vi "load_manual.vi"(8 "error in (no error)":errorcluster) -> (0 "error out":errorcluster, 2 "replaced_action(s)":bool, 3 "manual_actions out":variant)   [LabVIEW 2015, in "example_02.lvlib"]
doc: "load_manual.vi will assign manual steps as variant attributes to an empty variant. An indicator is provided if actions are replaced (e.g. a duplicate key)."
uses:
  example_02.lvlib
  <userlib>/antonio-alexander/lv-recipe-machine/public/_controls/step.ctl
  <userlib>/antonio-alexander/lv-recipe-machine/public/_controls/vi_reference_type.ctl
  _controls/steps_actions.ctl
  <userlib>/antonio-alexander/lv-recipe-machine/public/_controls/vi_reference_manual_action.ctl
  <userlib>/antonio-alexander/lv-recipe-machine/lv-recipe-machine.lvlib
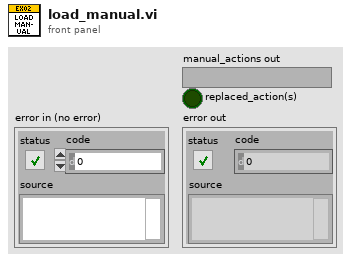
[diagram p1: front panel]
types:
  T1 = typedef "lv-recipe-machine.lvlib/vi_reference_type.ctl" = enum16{"<vi_reference_type>", "manual_action", "auto_step", "auto_criteria", "auto_transition", "auto_launcher", "<null>"}
  T2 = typedef "lv-recipe-machine.lvlib/step.ctl" = cluster{"name":string, "vi_reference":variant}
  T3 = typedef "lv-recipe-machine.lvlib/vi_reference_manual_action.ctl" = refnum<vi>
  T4 = typedef "example_02.lvlib/steps_actions.ctl" = enum16{"<steps_actions>", "auto_initialize", "auto_first_name", "auto_last_name", "criteria_", "transition", "launch_", "<null>"}
  T5 = cluster{"vi_reference_type":T1, "manual_action":T3}
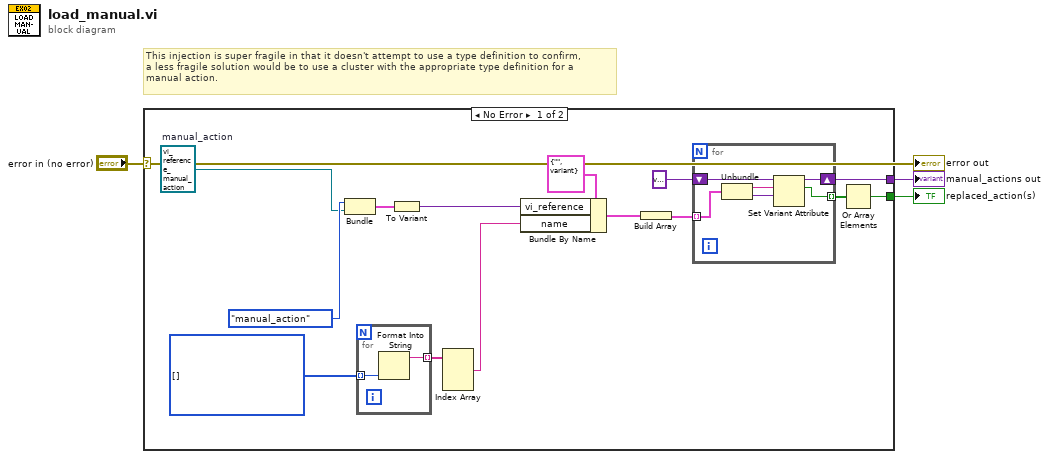
[diagram p0: block diagram]
diagram:
  # "This injection is super fragile in that it doesn't attempt to use a type definition to confirm,\na less fragile solution would be to use a cluster with the appropriate type definition for a\nmanual action."
  n1 = case shown="No Error" "error in (no error)" {
    tunnel: [w17 _] -> w3
    tunnel: [w14 _] -> w2
    frame No Error {
      w6 = T3 refnum  # manual_action
      w9 = T4[] [] items=["<steps_actions>", "auto_initialize", "auto_first_name", "auto_last_name", "criteria_", "transition", "launch_", "<null>"]
      n2 = Bundle("vi_reference_type"=vi_reference_type."manual_action", "manual_action"=w6) -> (w11:T5)  [unwired: 1 in]
      n3 = for {
        tunnel: w9 -> [w19] mode=indexing
        tunnel: [w18] -> w8 mode=indexing
        n4 = Format Into String(w19) -> (resulting string=w18:string)  [unwired: 3 in, 1 out]
      }
      n5 = To Variant(anything=w11) -> (Variant=w12:variant)
      n6 = Index Array(array=w8) -> (element #1=w7:string)  [unwired: 3 in, 2 out]
      n7 = Bundle By Name(cluster=T2 {"name"="", "vi_reference"=variant(refnum<vi> refnum)} ("step"), "vi_reference"=w12, "name"=w7) -> (w4:T2)
      n8 = Build Array(w4) -> (w16:T2[])
      n9 = for {
        tunnel: w16 -> [w23] mode=indexing
        shift-right: [w24] -> w17
        shift-left: variant ("manual_actions in") -> [w25]
        tunnel: [w21] -> w13 mode=indexing
        n10 = Unbundle(w23) -> ("name"=w22:string, "vi_reference"=w20:variant)
        n11 = Set Variant Attribute(Variant=w25, name=w22, value=w20) -> (Variant out=w24:variant, replaced=w21:bool)  [unwired: 1 in, 1 out]
      }
      n12 = Or Array Elements(Boolean array=w13) -> (logical OR=w14:bool)
    }
    frame Error {
    }
  }
  "manual_actions out" <- w3
  "replaced_action(s)" <- w2
  "error out" <- "error in (no error)"
